vi "Chat Launcher.vi"() -> ()   [LabVIEW 2020, in "Simple Chat.lvlib"]
uses:
  Simple Chat.lvlib
  Simple Chat/Simple Chat.lvclass
  C:/Program Files/National Instruments/LabVIEW 2020/vi.lib/ActorFramework/Actor/Actor.lvclass
  <vilib>/ActorFramework/Message Enqueuer/Message Enqueuer.lvclass/Message Enqueuer.ctl
  <vilib>/ActorFramework/Message Enqueuer/Enqueue.vi
  <vilib>/ActorFramework/Stop Msg/Stop Msg.lvclass
  C:/Program Files/National Instruments/LabVIEW 2020/vi.lib/ActorFramework/Message/Message.lvclass
  Actor Pub Sub Channels/Helpers/Get Topic Enqueuer.vi
  <vilib>/ActorFramework/Message Priority Queue/Priority Enqueue.vi
  <vilib>/ActorFramework/Actor/Actor.lvclass
  Actor Pub Sub Channels/Actor Pub Sub Channels.lvlib
panel:
  in  "stop":bool
  in  "Boolean":bool
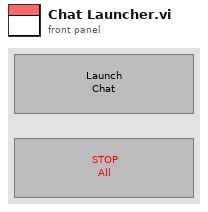
[diagram p1: front panel]
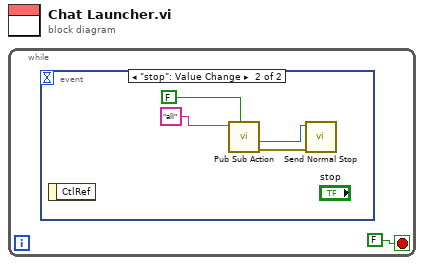
[diagram p0: block diagram]
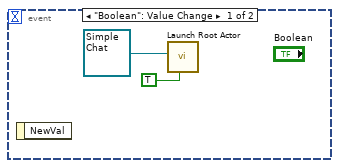
[diagram p2: hidden frame]
diagram:
  n1 = while {
    stop <- FALSE stop-if-true
    n2 = event shown="[1] \"stop\": Value Change" {
      selector: _ -> [_ _]
      dyn-events: _ -> [_ _]
      timeout: _ -> [_ _]
      event "Boolean": Value Change {
        n3 = event-data() -> ()  [unwired: 1 in, 1 out]
        n4 = call <vilib>:"Launch Root Actor.vi"("Open Actor Core front panel? (F)"=TRUE, "Actor"=refnum<class "Simple Chat.lvclass"> refnum ("Simple Chat.lvlib:Simple Chat.lvclass")) -> ()  [unwired: 8 in, 2 out]
      }
      event "stop": Value Change {
        n5 = event-data() -> ()  [unwired: 1 in, 1 out]
        n6 = call-poly "Pub Sub Action.vi"("Create if not exist? (T)"=FALSE, "Topic"="all") -> ("error out"=w5:errorcluster, "Topic Enqueuer"=w6:refnum<class "Message Enqueuer.lvclass">)  [unwired: 6 in, 2 out]
        n7 = call <vilib>:"Send Normal Stop.vi"("error in (no error)"=w5, "Message Enqueuer"=w6) -> ()  [unwired: 9 in, 1 out]
      }
    }
  }
